vi "Variant_to_Waveform.vi"(8 "Error in":errorcluster, 11 "Value (in)":variant) -> (0 "Error out":errorcluster, 2 "Value (string)":string, 3 "Value (out)":waveform(dbl))   [LabVIEW 2012]
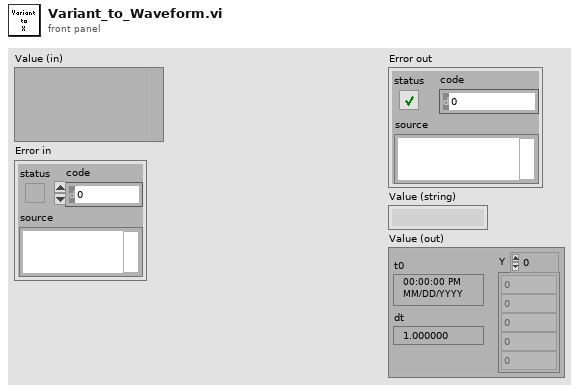
[diagram p1: front panel]
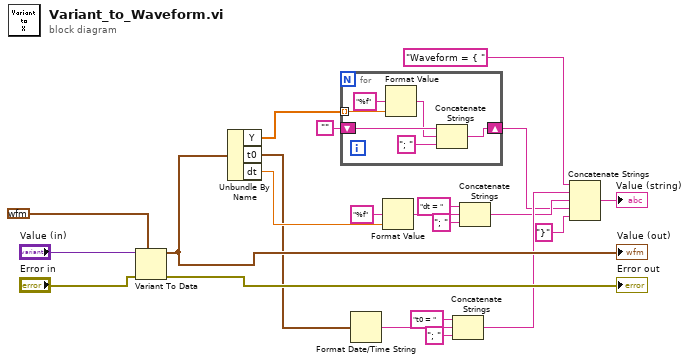
[diagram p0: block diagram]
diagram:
  n1 = Variant To Data(error in="Error in", type=waveform(dbl) {"t0"=timestamp(0 s since 1904-01-01), "dt"=1.0, "Y"=[]} ("Waveform"), Variant="Value (in)") -> (data=w19:waveform(dbl), error out=→"Error out":errorcluster)
  "Value (out)" <- w19
  n2 = Unbundle By Name(w19) -> ("Y"=w17:dbl[], "t0"=w11:timestamp, "dt"=w15:dbl)
  n3 = for {
    tunnel: w17 -> [w28] mode=indexing
    shift-right: [w25] -> w2
    shift-left: "" -> [w26]
    n4 = Format Value(format string="%f", value (0)=w28) -> (output string=w24:string)  [unwired: 1 in]
    n5 = Concatenate Strings(w26, w24, "; " ("string")) -> (w25:string)
  }
  n6 = Format Date/Time String(seconds (now)=w11) -> (date/time string=w8:string)  [unwired: 2 in]
  n7 = Format Value(format string="%f", value (0)=w15) -> (output string=w14:string)  [unwired: 1 in]
  n8 = Concatenate Strings("t0 = " ("string"), w8, "; " ("string")) -> (w4:string)
  n9 = Concatenate Strings("dt = " ("string"), w14, "; " ("string")) -> (w3:string)
  n10 = Concatenate Strings("Waveform = { " ("string"), w4, w3, w2, "}" ("string")) -> (→"Value (string)":string)
